vi "MS_Comm_to_Var_Analog.vi"(9 "Array":dbl[](array[numeric]), 11 "Boolean":bool) -> ()   [LabVIEW 2016, in "DNP3_Master_Station_MGCC.lvlib"]
uses:
  DNP3_Master_Station_MGCC.lvlib
  <vilib>/Utility/file.llb/Read Delimited Spreadsheet (string).vi
panel:
  out "element":refnum<k21>
  out "subarray":string[](array[string])
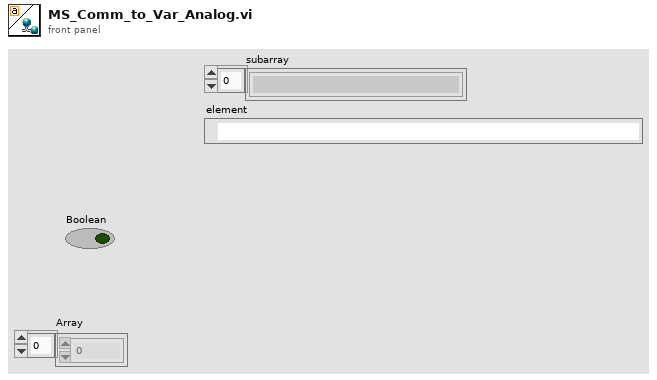
[diagram p1: front panel]
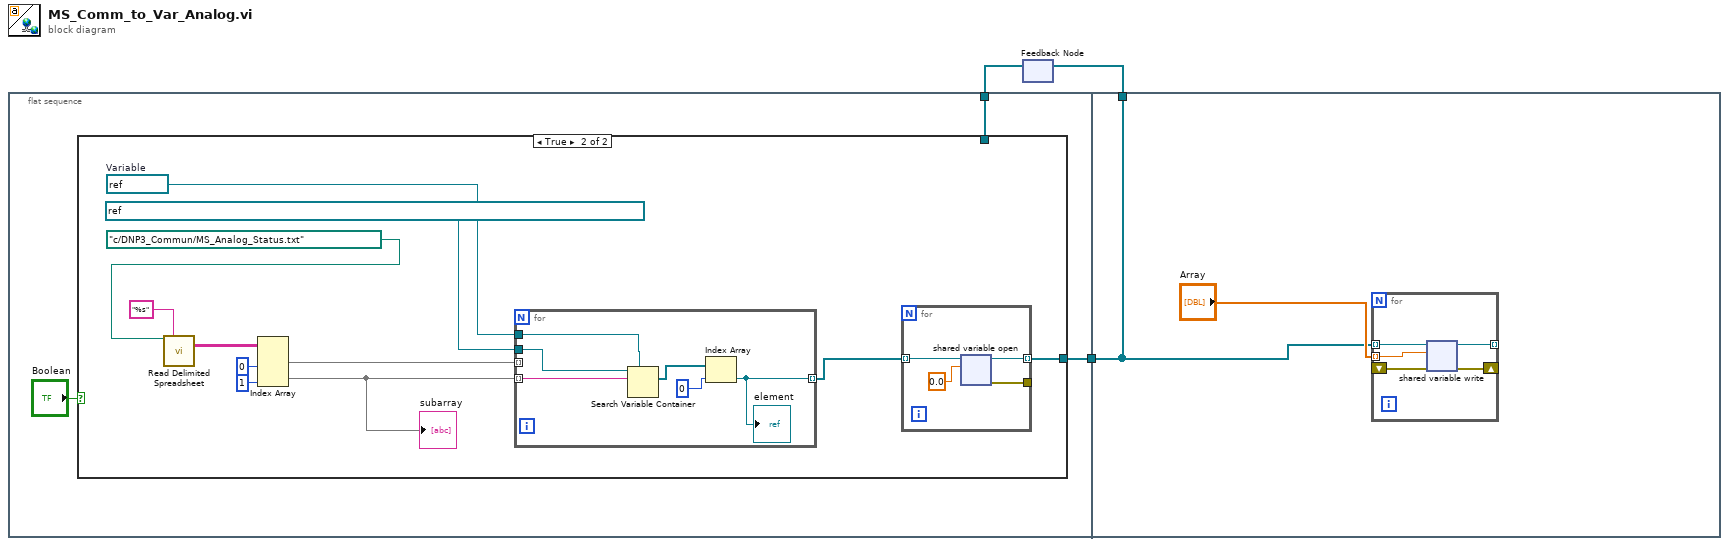
[diagram p0: block diagram]
diagram:
  n1 = flat-sequence {
    tunnel: [w6] -> w3
    tunnel: w1 -> [w4]
    tunnel: w3 -> [w29]
    tunnel: [w29] -> w2
    frame #0 {
      n2 = case shown="True" "Boolean" {
        tunnel: [w7 w8] -> w6
        tunnel: w4 -> [w7 _]
        frame False {
        }
        frame True {
          w10 = refnum<k21> refnum  # Variable
          n3 = call-poly <vilib>:"Read Delimited Spreadsheet.vi"("file path (dialog if empty)"=path "c:/DNP3_Commun/MS_Analog_Status.txt" ("file path (use dialog)"), "format (%s)"="%s") -> ("all rows"=w14:string[][])  [unwired: 8 in, 5 out]
          n4 = Index Array(array=w14, index (col) #1=0 ("disabled index (col)"), index (col) #2=1 ("index (col)")) -> (element #1=w17:string[], element #2=w18:string[])  [unwired: 2 in]
          "subarray" <- w18
          n5 = for {
            tunnel: w10 -> [w26]
            tunnel: refnum<k21> "ni.var.psp://mgcc/DNP3_Master_Station_MGCC/DNP3_Master_Data_Variables/MS_Analog_Status" ("container refnum in") -> [w25]
            tunnel: w17 -> [_] mode=indexing
            tunnel: w18 -> [w24] mode=indexing
            tunnel: [w23] -> w9 mode=indexing
            n6 = Search Variable Container(7:w26, 10:w24, 11:w25) -> (2:w28:refnum<k21>[])  [unwired: 3 in, 2 out]
            n7 = Index Array(array=w28, index=0) -> (element=w23:refnum<k21>)
            "element" <- w23
          }
          n8 = for {
            tunnel: [w22] -> w8 mode=indexing
            tunnel: [w21] -> _
            tunnel: w9 -> [w19] mode=indexing
            n9 = shared-variable-open(w19, 0.0) -> (w22:refnum<k21>, w21:errorcluster)  [unwired: 2 in]
          }
        }
      }
    }
    frame #1 {
      n10 = for {
        shift-right: [w34] -> _
        shift-left: _ -> [w35]
        tunnel: "Array" -> [w33] mode=indexing
        tunnel: w29 -> [w32] mode=indexing
        tunnel: [w31] -> _ mode=indexing
        n11 = shared-variable-write(w32, w35, w33) -> (w31:refnum<k21>, w34:errorcluster)
      }
    }
  }
  n12 = feedback-in #1(w2) -> ()
  n13 = feedback #1() -> (w1:refnum<k21>[])  [unwired: 1 in]
